vi "Cleanup Uplink.vi"(10 "Input String":string) -> (2 "Output String":string)   [LabVIEW 2010]
doc: "This VI removes all blank lines and all lines that begin with \"-- PULSE\" from the input string and outputs the resulting string to the Output String indicator."
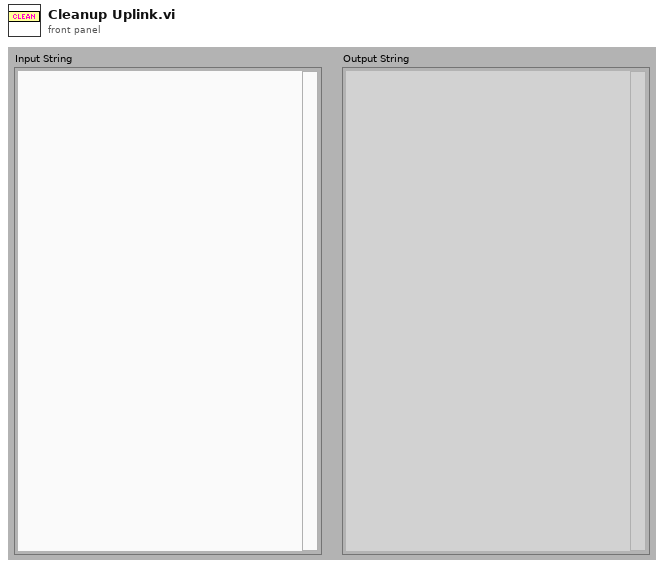
[diagram p1: front panel]
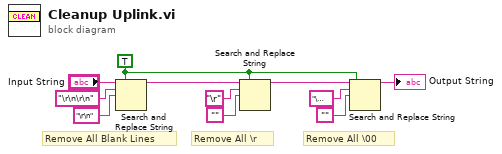
[diagram p0: block diagram]
diagram:
  w2 = TRUE ("replace all? (F)")
  # "Remove All \\00"
  # "Remove All \\r"
  # "Remove All Blank Lines"
  n1 = Search and Replace String(replace all?=w2, input string="Input String", search string="\r\n\r\n", replace string="\r\n" ("search string")) -> (result string=w8:string)  [unwired: 4 in, 3 out]
  n2 = Search and Replace String(replace all?=w2, input string=w8, search string="\r", replace string="" ("search string")) -> (result string=w3:string)  [unwired: 4 in, 3 out]
  n3 = Search and Replace String(replace all?=w2, input string=w3, search string="\u0000", replace string="" ("search string")) -> (result string=→"Output String":string)  [unwired: 4 in, 3 out]
